vi "Phasor Compute SEPL v2.vi"(6 "Tick Length (0.02)":dbl=0.02, 8 "Error In":errorcluster, 9 "Compute Lifetime/Fraction Array":bool, 11 "Phasor Parameters":T4={"Display Parameters"={"# Points"=0, "Ramp Type"=enum."Linear", "Type of Series"=enum."1-Exp Decays", "Min tau"=0.0, "Max tau"=0.0, "Include 0"=FALSE, "Include Infinity"=FALSE}, "Phasor Parameters"={"Harmonic Frequency"=0.0, "Use f* = 1/D Frequency"=FALSE, "Calibrated Phasor"=FALSE, "Calibration Lifetime"=1e-09, "Phasor Calculation"=enum."Direct Sum", "SEPL Type"=enum."UC", "# Gates"=1.0, "Square Gate Width"=1e-09, "Show Ticks"=FALSE}, "Decay & IRF Parameters"={"Lifetime"=0.0, "IRF Offset"=0.0, "IRF Period"=0.0, "Normalized Decays"=FALSE, "IRF Model"=enum."Dirac", "IRF Parameter 1"=0.0}, "Gate Parameters"={"First Gate Start"=0.0, "Use Gate Center"=FALSE, "Gate Width"=0.0, "Gate Step"=0.0, "# Gates"=0.0, "Gate Type"=enum."Square", "Edge Width"=0.0, "Top Slope"=0.0, "Reversed Sawtooth?"=FALSE, "Analytical Computation"=FALSE, "Integration"=enum."Item 0", "Tolerance"=1.0, "# Steps"=1.0, "Type of User-defined Function"=enum."Gate", "Use Gate Step"=FALSE}, "Detector Parameters"={"Frames/Image"=0, "Gates/Frame"=0, "Bits/Frame"=0, "Multiplicity"=0, "Incident Signal"=0.0, "Poisson Signal"=FALSE}} {"Detector Parameters"."Frames/Image" min=1; "Detector Parameters"."Multiplicity" min=0; "Detector Parameters"."Bits/Frame" min=1; "Detector Parameters"."Gates/Frame" min=1; "Gate Parameters"."# Steps" min=0.0; "Gate Parameters"."Tolerance" min=0.0; "Gate Parameters"."Top Slope" min=0.0; "Gate Parameters"."Edge Width" min=0.0; "Gate Parameters"."Gate Step" min=0.0; "Gate Parameters"."# Gates" min=0.0 step=1.0; "Gate Parameters"."Gate Width" min=0.0; "Decay & IRF Parameters"."Lifetime" min=0.0; "Decay & IRF Parameters"."IRF Period" min=0.0; "Phasor Parameters"."Square Gate Width" min=0.0; "Phasor Parameters"."# Gates" min=0.0; "Phasor Parameters"."Calibration Lifetime" min=0.0; "Phasor Parameters"."Harmonic Frequency" min=0.0; "Display Parameters"."Min tau" min=0.0; "Display Parameters"."Max tau" min=0.0; "Display Parameters"."# Points" min=1 step=1}) -> (0 "Error Out":errorcluster, 1 "Plot Name":string, 2 "Plot Metadata":T3={"Lifetime/Fraction Array"=[], "Phasor Explorer Parameters"={"Display Parameters"={"# Points"=0, "Ramp Type"=enum."Linear", "Type of Series"=enum."1-Exp Decays", "Min tau"=0.0, "Max tau"=0.0, "Include 0"=FALSE, "Include Infinity"=FALSE}, "Phasor Parameters"={"Harmonic Frequency"=0.0, "Use f* = 1/D Frequency"=FALSE, "Calibrated Phasor"=FALSE, "Calibration Lifetime"=1e-09, "Phasor Calculation"=enum."Direct Sum", "SEPL Type"=enum."UC", "# Gates"=1.0, "Square Gate Width"=1e-09, "Show Ticks"=FALSE}, "Decay & IRF Parameters"={"Lifetime"=0.0, "IRF Offset"=0.0, "IRF Period"=0.0, "Normalized Decays"=FALSE, "IRF Model"=enum."Dirac", "IRF Parameter 1"=0.0}, "Gate Parameters"={"First Gate Start"=0.0, "Use Gate Center"=FALSE, "Gate Width"=0.0, "Gate Step"=0.0, "# Gates"=0.0, "Gate Type"=enum."Square", "Edge Width"=0.0, "Top Slope"=0.0, "Reversed Sawtooth?"=FALSE, "Analytical Computation"=FALSE, "Integration"=enum."Item 0", "Tolerance"=1.0, "# Steps"=1.0, "Type of User-defined Function"=enum."Gate", "Use Gate Step"=FALSE}, "Detector Parameters"={"Frames/Image"=0, "Gates/Frame"=0, "Bits/Frame"=0, "Multiplicity"=0, "Incident Signal"=0.0, "Poisson Signal"=FALSE}}, "Phase Lifetimes"=[], "Modulus Lifetimes"=[]} {"Phasor Explorer Parameters"."Detector Parameters"."Frames/Image" min=1; "Phasor Explorer Parameters"."Detector Parameters"."Multiplicity" min=0; "Phasor Explorer Parameters"."Detector Parameters"."Bits/Frame" min=1; "Phasor Explorer Parameters"."Detector Parameters"."Gates/Frame" min=1; "Phasor Explorer Parameters"."Gate Parameters"."# Steps" min=0.0; "Phasor Explorer Parameters"."Gate Parameters"."Tolerance" min=0.0; "Phasor Explorer Parameters"."Gate Parameters"."Top Slope" min=0.0; "Phasor Explorer Parameters"."Gate Parameters"."Edge Width" min=0.0; "Phasor Explorer Parameters"."Gate Parameters"."Gate Step" min=0.0; "Phasor Explorer Parameters"."Gate Parameters"."# Gates" min=0.0 step=1.0; "Phasor Explorer Parameters"."Gate Parameters"."Gate Width" min=0.0; "Phasor Explorer Parameters"."Decay & IRF Parameters"."Lifetime" min=0.0; "Phasor Explorer Parameters"."Decay & IRF Parameters"."IRF Period" min=0.0; "Phasor Explorer Parameters"."Phasor Parameters"."Square Gate Width" min=0.0; "Phasor Explorer Parameters"."Phasor Parameters"."# Gates" min=0.0; "Phasor Explorer Parameters"."Phasor Parameters"."Calibration Lifetime" min=0.0; "Phasor Explorer Parameters"."Phasor Parameters"."Harmonic Frequency" min=0.0; "Phasor Explorer Parameters"."Display Parameters"."Min tau" min=0.0; "Phasor Explorer Parameters"."Display Parameters"."Max tau" min=0.0; "Phasor Explorer Parameters"."Display Parameters"."# Points" min=1 step=1}, 3 "Single Exponential Phasor Plot":cluster{"Array":dbl[], "Array":dbl[]}, 4 "Tick Label Data":T1[](array[typedef]), 5 "Phasor Calculation":T8, 7 "CPU (s)":dbl)   [LabVIEW 2021, in "Phasor.lvlib"]
uses:
  Phasor.lvlib
  Phasor SEPL Parameters.ctl
  Phasor Explorer Display Parameters.ctl
  Phasor Type of Series.ctl
  Phasor Explorer Phasor Parameters.ctl
  Phasor Calculation Type.ctl
  Phasor SEPL Type.ctl
  Phasor Explorer Decay Parameters.ctl
  Phasor IRF Model.ctl
  Phasor Explorer Gate Parameters.ctl
  Phasor Gate Type.ctl
  Phasor Type of User-defined Function.ctl
  Phasor Explorer Detector Parameters.ctl
  Phasor Explorer Phasor Plot Info.ctl
  Phasor SEPL Tick Data.ctl
  Phasor (g, s).ctl
  Phasor Calibration Data.ctl
  Phasor L_N[W] Parameters.ctl
  ba521b30-8e21-40a0-90b4-9632ea6a7fe5.vi
  Phasor Explorer.lvlib
  Time/Time.lvlib
panel:
  out "# Rejected Pairs":i32
  out "Lifetime/Fraction Array":dbl[](array[numeric])
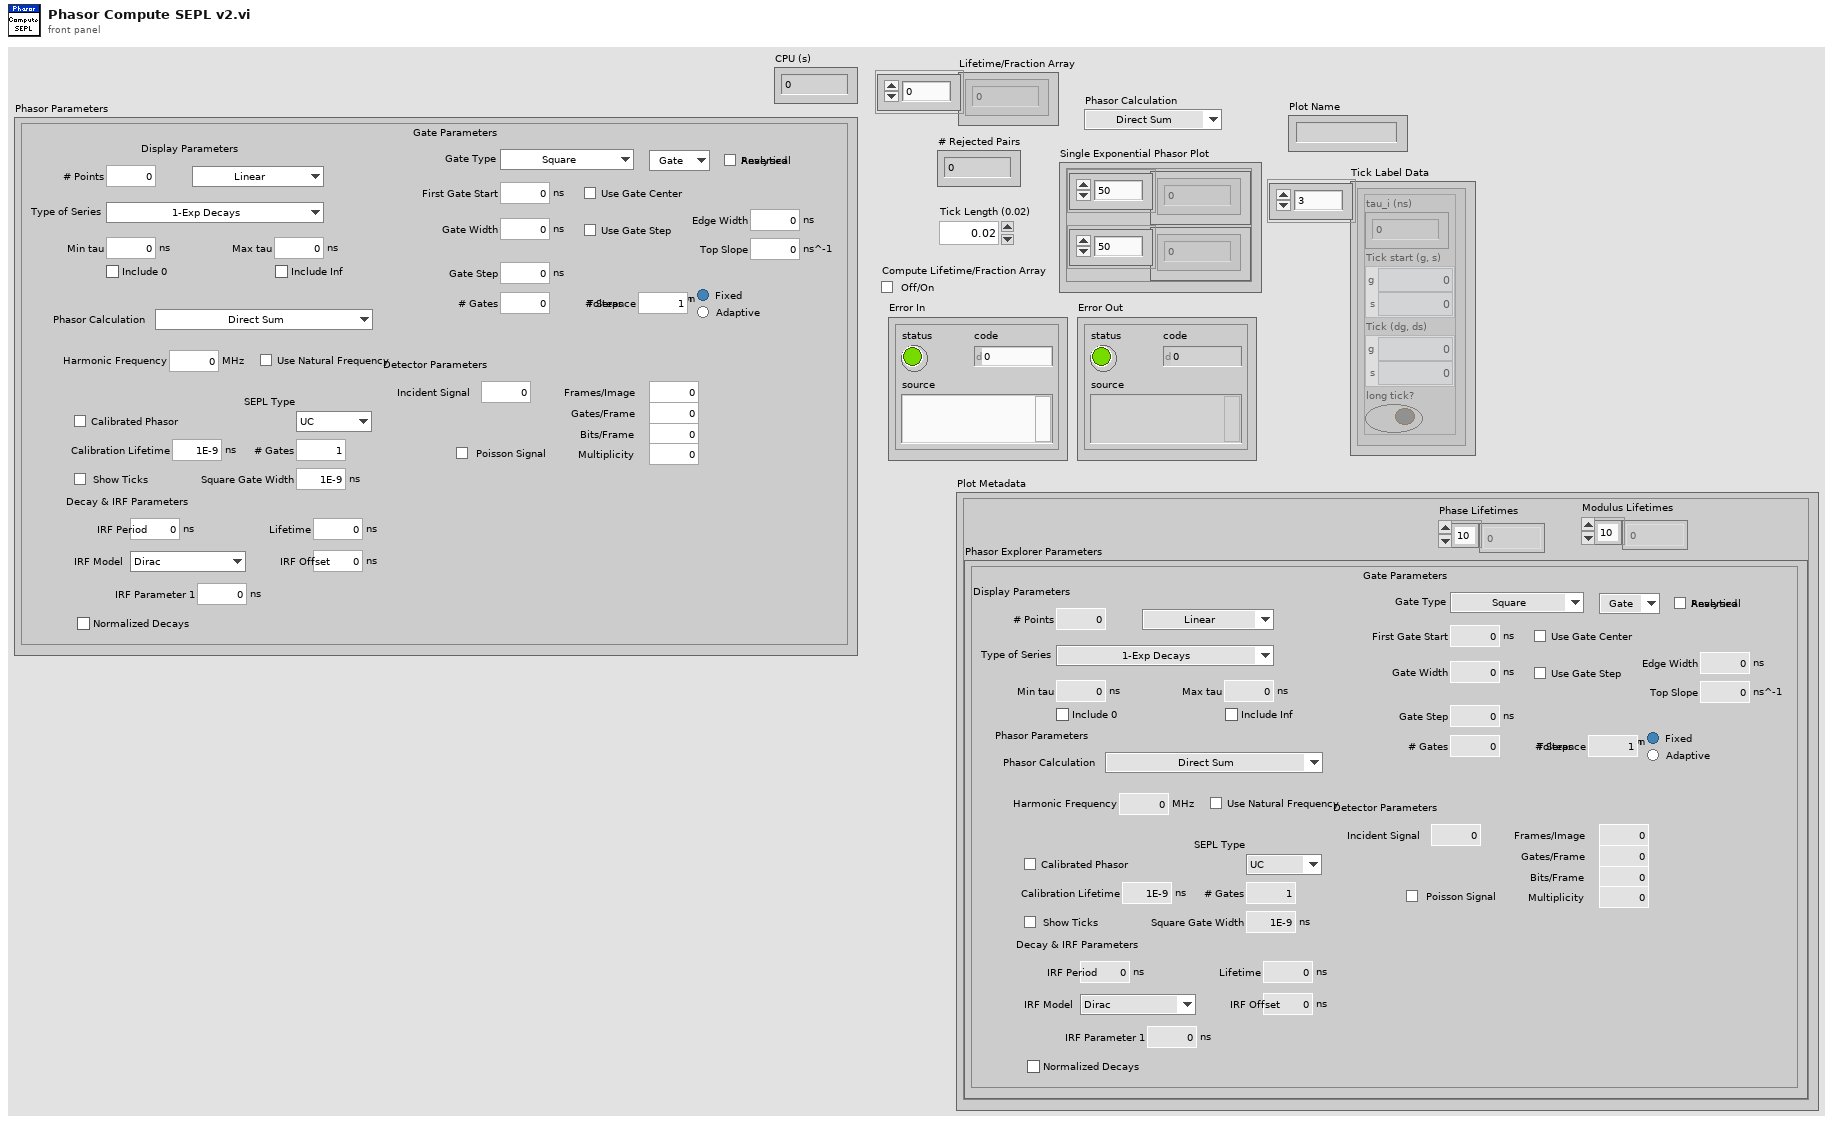
[diagram p1: front panel]
types:
  T1 = typedef "Phasor.lvlib/Phasor SEPL Tick Data.ctl" = cluster{"tau_i (ns)":dbl, "Tick start (g, s)":T2, "Tick (dg, ds)":T2, "long tick?":bool}
  T2 = typedef "Phasor.lvlib/Phasor (g, s).ctl" = cluster{"g":dbl, "s":dbl}
  T3 = typedef "Phasor Explorer.lvlib/Phasor Explorer Phasor Plot Info.ctl" = cluster{"Lifetime/Fraction Array":dbl[], "Phasor Explorer Parameters":T4, "Phase Lifetimes":dbl[], "Modulus Lifetimes":dbl[]}
  T4 = typedef "Phasor.lvlib/Phasor SEPL Parameters.ctl" = cluster{"Display Parameters":T5, "Phasor Parameters":T7, "Decay & IRF Parameters":T10, "Gate Parameters":T12, "Detector Parameters":T15}
  T5 = typedef "Phasor Explorer.lvlib/Phasor Explorer Display Parameters.ctl" = cluster{"# Points":i32, "Ramp Type":enum16{"Linear", "Logarithmic"}, "Type of Series":T6, "Min tau":dbl[unit], "Max tau":dbl[unit], "Include 0":bool, "Include Infinity":bool}
  T6 = typedef "Phasor.lvlib/Phasor Type of Series.ctl" = enum16{"1-Exp Decays", "Linear Combination of 1-Exp"}
  T7 = typedef "Phasor Explorer.lvlib/Phasor Explorer Phasor Parameters.ctl" = cluster{"Harmonic Frequency":dbl[unit], "Use f* = 1/D Frequency":bool, "Calibrated Phasor":bool, "Calibration Lifetime":dbl[unit], "Phasor Calculation":T8, "SEPL Type":T9, "# Gates":dbl, "Square Gate Width":dbl[unit], "Show Ticks":bool}
  T8 = typedef "Phasor.lvlib/Phasor Calculation Type.ctl" = enum16{"Direct Sum", "Analytical Formula"}
  T9 = typedef "Phasor.lvlib/Phasor SEPL Type.ctl" = enum16{"UC", "L_N", "L_N[W]", "L_X"}
  T10 = typedef "Phasor Explorer.lvlib/Phasor Explorer Decay Parameters.ctl" = cluster{"Lifetime":dbl[unit], "IRF Offset":dbl[unit], "IRF Period":dbl[unit], "Normalized Decays":bool, "IRF Model":T11, "IRF Parameter 1":dbl[unit]}
  T11 = typedef "Phasor.lvlib/Phasor IRF Model.ctl" = enum16{"Dirac", "Exponential"}
  T12 = typedef "Phasor Explorer.lvlib/Phasor Explorer Gate Parameters.ctl" = cluster{"First Gate Start":dbl[unit], "Use Gate Center":bool, "Gate Width":dbl[unit], "Gate Step":dbl[unit], "# Gates":dbl, "Gate Type":T13, "Edge Width":dbl[unit], "Top Slope":dbl[unit], "Reversed Sawtooth?":bool, "Analytical Computation":bool, "Integration":enum32{"Item 0", "Item 1"}, "Tolerance":dbl, "# Steps":dbl, "Type of User-defined Function":T14, "Use Gate Step":bool}
  T13 = typedef "Phasor.lvlib/Phasor Gate Type.ctl" = enum16{"Square", "Finite Edge Square", "Finite Edge, Tilted Top Square", "Triangle", "Sawtooth", "User-defined"}
  T14 = typedef "Phasor.lvlib/Phasor Type of User-defined Function.ctl" = enum16{"Gate", "IRF"}
  T15 = typedef "Phasor Explorer.lvlib/Phasor Explorer Detector Parameters.ctl" = cluster{"Frames/Image":i32, "Gates/Frame":i32, "Bits/Frame":i32, "Multiplicity":i32, "Incident Signal":dbl, "Poisson Signal":bool}
  T16 = typedef "Phasor.lvlib/Phasor L_N[W] Parameters.ctl" = cluster{"Laser Period":dbl[unit], "Gate Width":dbl[unit], "Gate Step":dbl[unit], "Harmonic frequency":dbl[unit], "IRF offset":dbl[unit], "# Gates":dbl}
  T17 = typedef "Phasor.lvlib/Phasor Calibration Data.ctl" = cluster{"jw":cxt, "Uncalibrated Phasor":cxt, "Calibrated Phasor":cxt, "Calibrated Phasor?":bool, "Calibration Lifetime":ext}
  T18 = typedef "Phasor.lvlib/Phasor Gate Definitions.ctl" = cluster{"First Gate: t1":ext, "Gate Width: W":ext, "Gate Step: d":ext, "# Gates: G":ext, "Use Gate Center":bool, "Frames/Image: F":i32, "Gates/Frame: L":i32, "Bits/Frame: q":i32, "Multiplicity: p":i32, "Gate Type":T13, "Gate Edge s":ext, "Gate Top Slope":ext, "Reversed Sawtooth?":bool, "Computation":bool, "User-defined Gate":T19, "Tolerance":ext, "Integration":enum32{"Item 0", "Item 1"}, "# Steps":ext, "Type of User-defined Function":enum32{"Gate", "IRF"}}
  T19 = typedef "XY Graph Add-Ons.lvlib/XY Plot Data.ctl" = cluster{"X Array":dbl[], "Y Array":dbl[]}
  T20 = typedef "Phasor.lvlib/Phasor Decay Definiton.ctl" = cluster{"offset: t0":ext, "period: T":ext, "lifetime: tau":ext, "Incident Signal: I":ext, "Normalized Decays":bool, "IRF Model":T11, "IRF Parameter 1":ext, "Poisson Signal":bool}
  T21 = cluster{"Numeric Control":ext, "Numeric Control":ext}
  T22 = cluster{"Calibrated g Array out":ext[], "Calibrated s Array out":ext[]}
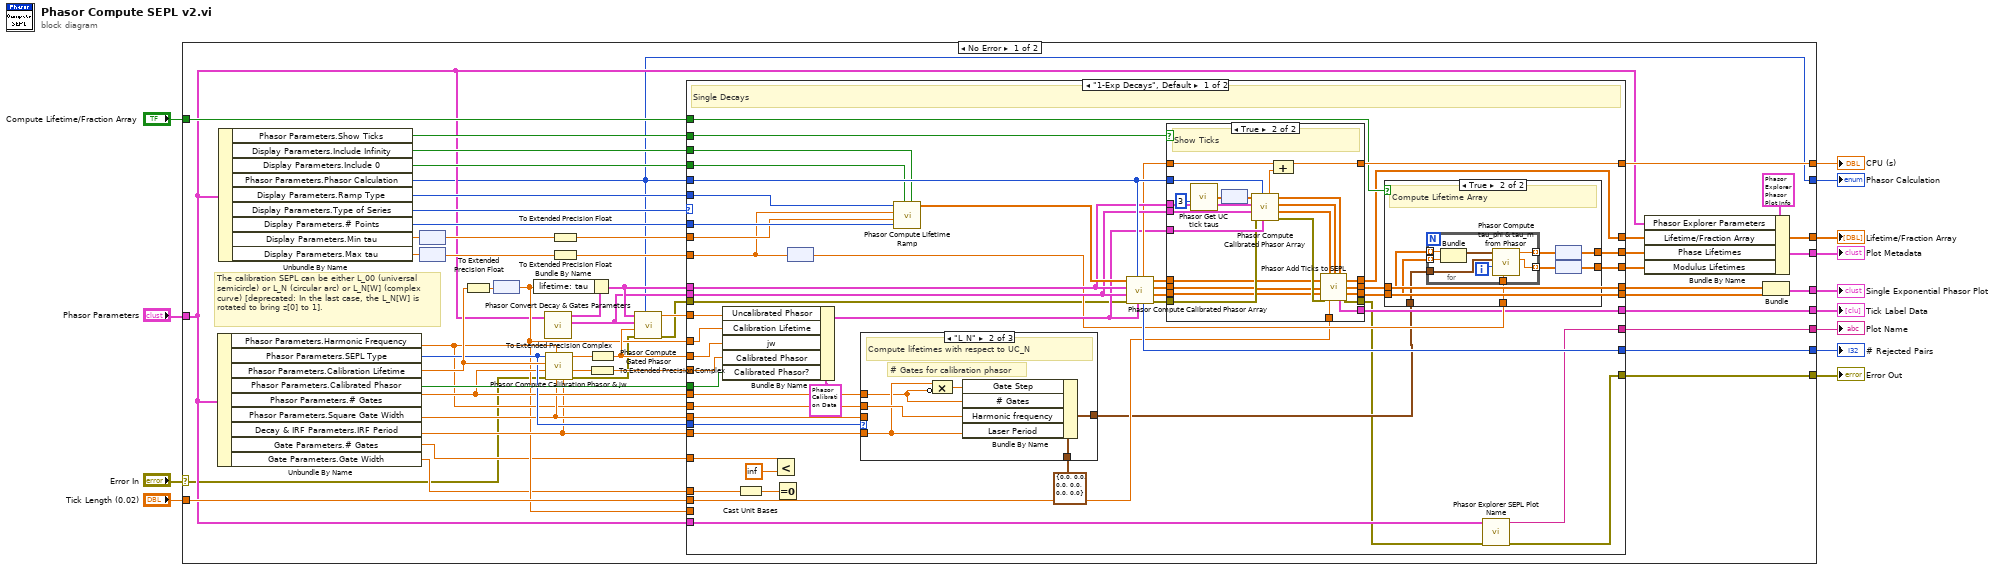
[diagram p0: block diagram]
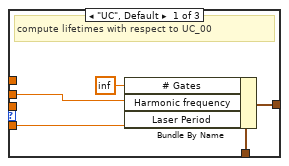
[diagram p4: hidden frame]
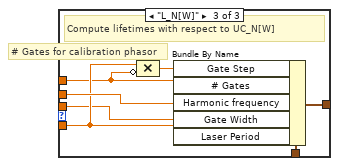
[diagram p5: hidden frame]
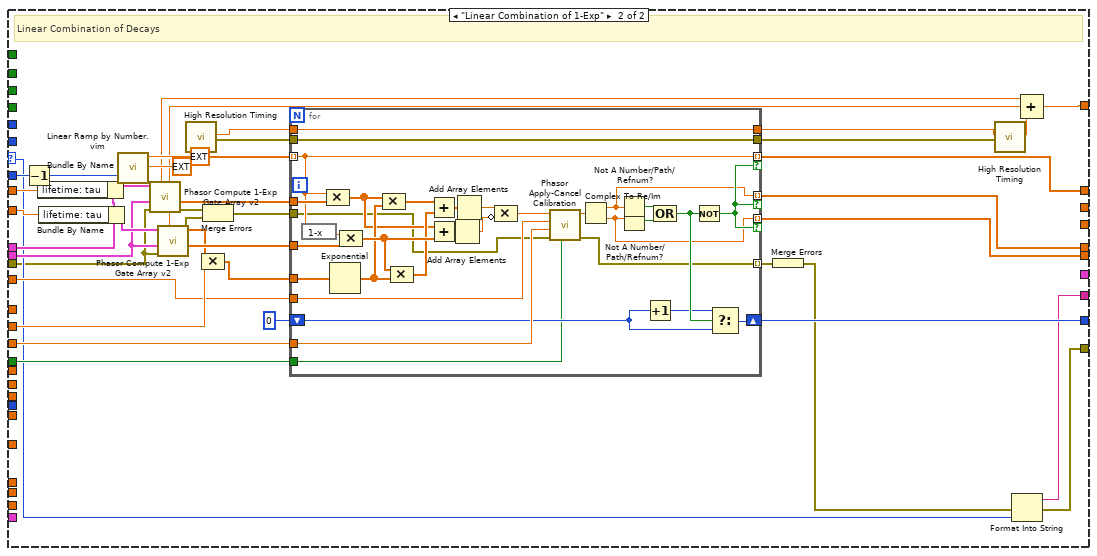
[diagram p6: hidden frame]
diagram:
  n1 = case shown="No Error" "Error In" {
    selector: "Error In" -> [w17 w251]
    tunnel: "Phasor Parameters" -> [w18 _]
    tunnel: [w58 _] -> w12
    tunnel: [w30 w251] -> w10
    tunnel: [w39 _] -> w9
    tunnel: [w14 _] -> w8
    tunnel: [w29 _] -> w7
    tunnel: [w45 _] -> w6
    tunnel: [w34 _] -> w5
    tunnel: [w32 _] -> w4
    tunnel: "Compute Lifetime/Fraction Array" -> [w28 _]
    tunnel: "Tick Length (0.02)" -> [w27 _]
    tunnel: [w26 _] -> w1
    frame No Error {
      # "The calibration SEPL can be either L_00 (universal semicircle) or L_N (circular arc) or L_N[W] (complex curve) [deprecated: In the last case, the L_N[W] is rotated to bring z[0] to 1]."
      n2 = Unbundle By Name(w18) -> ("Phasor Parameters.Harmonic Frequency"=w23:dbl[unit], "Phasor Parameters.SEPL Type"=w35:T9, "Phasor Parameters.Calibration Lifetime"=w41:dbl[unit], "Phasor Parameters.Calibrated Phasor"=w50:bool, "Phasor Parameters.# Gates"=w25:dbl, "Phasor Parameters.Square Gate Width"=w24:dbl[unit], "Decay & IRF Parameters.IRF Period"=w22:dbl[unit], "Gate Parameters.# Gates"=w20:dbl, "Gate Parameters.Gate Width"=w19:dbl[unit])
      n3 = Unbundle By Name(w18) -> ("Phasor Parameters.Show Ticks"=w33:bool, "Display Parameters.Include Infinity"=w48:bool, "Display Parameters.Include 0"=w49:bool, "Phasor Parameters.Phasor Calculation"=w14:T8, "Display Parameters.Ramp Type"=w57:enum16{"Linear", "Logarithmic"}, "Display Parameters.Type of Series"=w53:T6, "Display Parameters.# Points"=w31:i32, "Display Parameters.Min tau"=w59:dbl[unit], "Display Parameters.Max tau"=w64:dbl[unit])
      n4 = node(w59) -> (w55:dbl)
      n5 = node(w64) -> (w54:dbl)
      n6 = To Extended Precision Float(1:w41) -> (0:w43:ext[unit])
      n7 = node(w43) -> (w21:ext)
      n8 = call "Phasor Convert Decay & Gates Parameters.vi"("Phasor Parameters"=w18) -> ("Gates Definitions"=w51:T18, "Decay Definition"=w52:T20)  [unwired: 9 in]
      n9 = Bundle By Name(cluster=w52, "lifetime: tau"=w21) -> (w60:T20)
      n10 = call "Phasor Compute Calibration Phasor & jw.vi"("Laser Period"=w22, "Gate Width"=w24, "Harmonic frequency"=w23, "Error In"=w17, "# Gates"=w25, "Calibration Lifetime"=w41, "Calibration Phasor Type"=w35) -> ("Error Out"=w16:errorcluster, "z (tau_cal)"=w36:cdb, "i 2 pi f (GHz)"=w56:cdb)  [unwired: 2 in]
      n11 = To Extended Precision Float(1:w55) -> (0:w47:ext)
      n12 = To Extended Precision Float(1:w54) -> (0:w46:ext)
      n13 = To Extended Precision Complex(1:w36) -> (0:w44:cxt)
      n14 = To Extended Precision Complex(1:w56) -> (0:w42:cxt)
      n15 = call "Phasor Compute Gated Phasor.vi"("Phasor Calculation Type"=w14, "Error In"=w16, "j 2 pi f"=w42, "Gates Definitions"=w51, "Decay Definition"=w60) -> ("Error Out"=w15:errorcluster, "phasor"=w61:cxt)  [unwired: 4 in, 1 out]
      n16 = case shown="\"1-Exp Decays\", Default" w53 {
        selector: w53 -> [_ w181]
        tunnel: [w89 w197] -> w63
        tunnel: [w88 w196] -> w62
        tunnel: w50 -> [w69 w205]
        tunnel: w61 -> [w114 w203]
        tunnel: w60 -> [w98 w217]
        tunnel: w51 -> [w97 w213]
        tunnel: w42 -> [w111 w207]
        tunnel: w44 -> [w113 w204]
        tunnel: w47 -> [w82 w218]
        tunnel: w46 -> [w81 w216]
        tunnel: w57 -> [w84 _]
        tunnel: w21 -> [w110 _]
        tunnel: w14 -> [w100 _]
        tunnel: [w71 w198] -> w39
        tunnel: [w65 w178] -> w30
        tunnel: w49 -> [w86 _]
        tunnel: w48 -> [w85 _]
        tunnel: [w108 w199] -> w45
        tunnel: [w106 _] -> w38
        tunnel: [w107 _] -> w37
        tunnel: w35 -> [w78 _]
        tunnel: w23 -> [w104 _]
        tunnel: w22 -> [w103 _]
        tunnel: w25 -> [w102 _]
        tunnel: [w95 w189] -> w34
        tunnel: w24 -> [w101 _]
        tunnel: w33 -> [w99 _]
        tunnel: w31 -> [w83 w184]
        tunnel: [w68 w182] -> w29
        tunnel: w28 -> [w80 _]
        tunnel: w27 -> [w75 _]
        tunnel: [w79 _] -> w26
        tunnel: w21 -> [_ _]
        tunnel: w20 -> [w77 _]
        tunnel: w19 -> [w73 _]
        tunnel: w18 -> [w70 _]
        tunnel: w15 -> [w67 w180]
        frame "1-Exp Decays", Default {
          # "Single Decays"
          n17 = Bundle By Name(cluster=T17 {"jw"=0.0+0.0i, "Uncalibrated Phasor"=0.0+0.0i, "Calibrated Phasor"=0.0+0.0i, "Calibrated Phasor?"=FALSE, "Calibration Lifetime"=0.0} ("output cluster"), "Uncalibrated Phasor"=w114, "Calibration Lifetime"=w110, "jw"=w111, "Calibrated Phasor"=w113, "Calibrated Phasor?"=w69) -> (w91:T17)
          n18 = Cast Unit Bases(0:w73) -> (2:w72:dbl)  [unwired: 1 in]
          n19 = Less?(x=w77, y=inf) -> ()  [unwired: 1 out]
          n20 = Equal To 0?(x=w72) -> ()  [unwired: 1 out]
          n21 = node(w81) -> (w87:ext[unit])
          n22 = case shown="\"L_N\"" w78 {
            tunnel: [w164 w170 w177] -> w74
            tunnel: T16 {"Laser Period"=0.0, "Gate Width"=0.0, "Gate Step"=0.0, "Harmonic frequency"=0.0, "IRF offset"=0.0, "# Gates"=0.0} ("Phasor UCN[W] Parameters") -> [w162 w169 w176]
            tunnel: w104 -> [w161 w168 w175]
            tunnel: w103 -> [w160 w167 w174]
            tunnel: w102 -> [_ w165 w172]
            tunnel: w101 -> [_ _ w171]
            frame "UC", Default {
              # "compute lifetimes with respect to UC_00"
              n23 = Bundle By Name(cluster=w162, "# Gates"=inf ("Gate Parameters.# Gates"), "Harmonic frequency"=w161, "Laser Period"=w160) -> (w164:T16)
            }
            frame "L_N" {
              # "# Gates for calibration phasor"
              # "Compute lifetimes with respect to UC_N"
              n24 = Compound Arithmetic op=MULTIPLY(w167, invert w165) -> (w166:dbl[unit])
              n25 = Bundle By Name(cluster=w169, "Gate Step"=w166, "# Gates"=w165, "Harmonic frequency"=w168, "Laser Period"=w167) -> (w170:T16)
            }
            frame "L_N[W]" {
              # "# Gates for calibration phasor"
              # "Compute lifetimes with respect to UC_N[W]"
              n26 = Compound Arithmetic op=MULTIPLY(w174, invert w172) -> (w173:dbl[unit])
              n27 = Bundle By Name(cluster=w176, "Gate Step"=w173, "# Gates"=w172, "Harmonic frequency"=w175, "Gate Width"=w171, "Laser Period"=w174) -> (w177:T16)
            }
          }
          n28 = call "Phasor Compute Lifetime Ramp.vi"("Include Infinity"=w85, "Include 0"=w86, "# Points"=w83, "Min Tau"=w82, "Max Tau"=w81, "Ramp Type"=w84) -> ("Lifetime Ramp"=w109:ext[])  [unwired: 5 in]
          n29 = call "Phasor Compute Calibrated Phasor Array.vi"("Phasor Calibration Data"=w91, "Phasor Calculation"=w100, "Error In"=w67, "Gates Definitions"=w97, "Decay Definition"=w98, "Lifetime Array"=w109) -> ("Error Out"=w90:errorcluster, "Calibrated s Array"=w92:ext[], "Calibrated g Array"=w93:ext[], "True Lifetime Array"=w94:ext[], "# Rejected Pairs"=w108:i32, "CPU (s)"=w96:dbl)
          n30 = case shown="True" w99 {
            tunnel: w100 -> [_ w159]
            tunnel: w98 -> [_ w158]
            tunnel: w97 -> [_ w157]
            tunnel: [w134 w148] -> w66
            tunnel: w96 -> [w135 w156]
            tunnel: [w135 w154] -> w95
            tunnel: w94 -> [w133 w146]
            tunnel: w93 -> [w132 w145]
            tunnel: w92 -> [w131 w144]
            tunnel: w91 -> [_ w151]
            tunnel: w90 -> [w134 w150]
            tunnel: [w133 w143] -> w71
            tunnel: [w132 w142] -> w89
            tunnel: [w131 w141] -> w88
            tunnel: w75 -> [_ w138]
            tunnel: [_ w137] -> w79
            frame False {
            }
            frame True {
              # "Show Ticks"
              n31 = call "Phasor Get UC tick taus.vi"("# Decades (4: 10 ps - 900 ns)"=3) -> ("Array of taus"=w153:dbl[unit][])  [unwired: 7 in]
              n32 = node(w153) -> (w152:dbl[])
              n33 = call "Phasor Compute Calibrated Phasor Array.vi"("Phasor Calibration Data"=w151, "Phasor Calculation"=w159, "Error In"=w150, "Gates Definitions"=w157, "Decay Definition"=w158, "Lifetime Array"=w152) -> ("Error Out"=w149:errorcluster, "Calibrated s Array"=w140:ext[], "Calibrated g Array"=w139:ext[], "True Lifetime Array"=w147:ext[], "CPU (s)"=w155:dbl)  [unwired: 1 out]
              n34 = Compound Arithmetic op=ADD(w156, w155) -> (w154:dbl)
              n35 = call "Phasor Add Ticks to SEPL.vi"("Ticks Calibrated s's"=w140, "Ticks Calibrated g's"=w139, "Ticks Lifetimes"=w147, "Lifetime Array in"=w146, "Calibrated g Array in"=w145, "Calibrated s Array in"=w144, "error in (no error)"=w149, "Tick Length"=w138) -> ("Lifetime Array out"=w143:ext[], "Calibrated g Array out"=w142:ext[], "Calibrated s Array out"=w141:ext[], "Tick Labels (g,s))"=w137:T1[], "error out"=w148:errorcluster)  [unwired: 3 in]
            }
          }
          n36 = case shown="True" w80 {
            tunnel: [_ w120] -> w107
            tunnel: [_ w119] -> w106
            tunnel: w74 -> [_ w118]
            tunnel: w89 -> [_ w117]
            tunnel: w88 -> [_ w116]
            tunnel: w87 -> [_ w115]
            frame False {
            }
            frame True {
              # "Compute Lifetime Array"
              n37 = for {
                tunnel: w115 -> [w124]
                tunnel: w118 -> [w125]
                tunnel: w117 -> [w128] mode=indexing
                tunnel: w116 -> [w127] mode=indexing
                tunnel: [w130] -> w122 mode=indexing
                tunnel: [w129] -> w121 mode=indexing
                i -> [w123]
                n38 = Bundle("Numeric Control"=w128, "Numeric Control"=w127) -> (w126:T21)  [unwired: 1 in]
                n39 = call "Phasor Compute tau_phi & tau_m from Phasor.vi"("max tau"=w124, "Call # (0)"=w123, "Phasor L_N[W] Parameters"=w125, "Phasor"=w126) -> ("tau_m"=w130:dbl[unit], "tau_ph"=w129:dbl[unit])  [unwired: 5 in, 1 out]
              }
              n40 = node(w121) -> (w120:dbl[])
              n41 = node(w122) -> (w119:dbl[])
            }
          }
          n42 = call "Phasor Explorer SEPL Plot Name.vi"("Error In"=w66, "Phasor Parameters"=w70) -> ("Error Out"=w65:errorcluster, "SEPL Plot Name"=w68:string)  [unwired: 8 in]
        }
        frame "Linear Combination of 1-Exp" {
          # "Linear Combination of Decays"
          n43 = Decrement(x=w184) -> (x-1=w183:i32)
          n44 = Bundle By Name(cluster=w217, "lifetime: tau"=w218) -> (w215:T20)
          n45 = Bundle By Name(cluster=w217, "lifetime: tau"=w216) -> (w214:T20)
          n46 = call "Linear Ramp by Number.vim"("# Steps (1)"=w183, "End (1)"=ext 1.0 ("Max"), "Start (0)"=ext 0.0 ("Min")) -> ("Ramp"=w200:ext[])  [unwired: 6 in, 2 out]
          n47 = call "Phasor Compute 1-Exp Gate Array v2.vi"("Error In"=w180, "Gates Definitions"=w213, "Decay Definition"=w215) -> ("Error Out"=w202:errorcluster, "Gate Image Array"=w210:ext[], "CPU (s)"=w188:dbl)  [unwired: 4 in, 2 out]
          n48 = call "Phasor Compute 1-Exp Gate Array v2.vi"("Error In"=w180, "Gates Definitions"=w213, "Decay Definition"=w214) -> ("Error Out"=w201:errorcluster, "Gate Image Array"=w209:ext[], "t Array"=w208:ext[], "CPU (s)"=w187:dbl)  [unwired: 4 in, 1 out]
          n49 = call "High Resolution Timing.vi"() -> ("elapsed (relative) seconds"=w192:dbl, "Error Out"=w194:errorcluster)  [unwired: 17 in, 1 out]
          n50 = Compound Arithmetic op=MULTIPLY(w208, w207) -> (w206:cxt[])
          n51 = Merge Errors(w202, w201) -> (w186:errorcluster)
          n52 = for {
            tunnel: w210 -> [w250]
            tunnel: w209 -> [w249]
            tunnel: w200 -> [w230] mode=indexing
            tunnel: w206 -> [w248]
            tunnel: [w226] -> w196 mode=indexing if=w229
            tunnel: [w225] -> w197 mode=indexing if=w229
            tunnel: w205 -> [w221]
            tunnel: w204 -> [w235]
            tunnel: w203 -> [w234]
            tunnel: [w230] -> w198 mode=indexing if=w229
            shift-right: [w228] -> w199
            shift-left: 0 -> [w227]
            tunnel: w194 -> [w223]
            tunnel: [w223] -> w193
            tunnel: w192 -> [w222]
            tunnel: [w222] -> w191
            tunnel: w186 -> [w220]
            tunnel: [w219] -> w185 mode=indexing
            n53 = expression code="1-x"(w230) -> (w245:ext)
            n54 = Compound Arithmetic op=MULTIPLY(w230, w250) -> (w240:ext[])
            n55 = Exponential(1:w248) -> (0:w246:cxt[])
            n56 = Compound Arithmetic op=MULTIPLY(w245, w249) -> (w247:ext[])
            n57 = Compound Arithmetic op=MULTIPLY(w240, w246) -> (w244:cxt[])
            n58 = Compound Arithmetic op=MULTIPLY(w247, w246) -> (w243:cxt[])
            n59 = Add(x=w244, y=w243) -> (x+y=w242:cxt[])
            n60 = Add(x=w240, y=w247) -> (x+y=w241:ext[])
            n61 = Add Array Elements(numeric array=w241) -> (sum=w238:ext)
            n62 = Add Array Elements(numeric array=w242) -> (sum=w239:cxt)
            n63 = Compound Arithmetic op=MULTIPLY(w239, invert w238) -> (w237:cxt)
            n64 = call "Phasor Apply-Cancel Calibration.vi"("Calibrated Phasor"=w221, "Error In"=w220, "Target Phasor"=w235, "Calibration Phasor"=w234, "Phasor in"=w237) -> ("Error Out"=w219:errorcluster, "Phasor out"=w236:cxt)  [unwired: 5 in]
            n65 = Complex To Re/Im(x + iy=w236) -> (x=w225:ext, y=w226:ext)
            n66 = Not A Number/Path/Refnum?(number/path/refnum=w225) -> (NaN/Path/Refnum?=w224:bool)
            n67 = Not A Number/Path/Refnum?(number/path/refnum=w226) -> (NaN/Path/Refnum?=w233:bool)
            n68 = Increment(x=w227) -> (x+1=w231:i32)
            n69 = Compound Arithmetic op=OR(w224, w233) -> (w232:bool)
            n70 = Not(x=w232) -> (.not. x?=w229:bool)
            n71 = Select(t=w231, s=w232, f=w227) -> (s? t:f=w228:i32)
          }
          n72 = Merge Errors(w185) -> (w179:errorcluster)
          n73 = call "High Resolution Timing.vi"("relative seconds (NaN)"=w191, "Error In"=w193) -> ("elapsed (relative) seconds"=w190:dbl)  [unwired: 15 in, 2 out]
          n74 = Format Into String(error in=w179, w181) -> (resulting string=w182:string, error out=w178:errorcluster)  [unwired: 2 in]
          n75 = Compound Arithmetic op=ADD(w188, w187, w190) -> (w189:dbl)
        }
      }
      n76 = Bundle By Name(cluster=T3 {"Lifetime/Fraction Array"=[], "Phasor Explorer Parameters"={"Display Parameters"={"# Points"=0, "Ramp Type"=enum."Linear", "Type of Series"=enum."1-Exp Decays", "Min tau"=0.0, "Max tau"=0.0, "Include 0"=FALSE, "Include Infinity"=FALSE}, "Phasor Parameters"={"Harmonic Frequency"=0.0, "Use f* = 1/D Frequency"=FALSE, "Calibrated Phasor"=FALSE, "Calibration Lifetime"=1e-09, "Phasor Calculation"=enum."Direct Sum", "SEPL Type"=enum."UC", "# Gates"=1.0, "Square Gate Width"=1e-09, "Show Ticks"=FALSE}, "Decay & IRF Parameters"={"Lifetime"=0.0, "IRF Offset"=0.0, "IRF Period"=0.0, "Normalized Decays"=FALSE, "IRF Model"=enum."Dirac", "IRF Parameter 1"=0.0}, "Gate Parameters"={"First Gate Start"=0.0, "Use Gate Center"=FALSE, "Gate Width"=0.0, "Gate Step"=0.0, "# Gates"=0.0, "Gate Type"=enum."Square", "Edge Width"=0.0, "Top Slope"=0.0, "Reversed Sawtooth?"=FALSE, "Analytical Computation"=FALSE, "Integration"=enum."Item 0", "Tolerance"=1.0, "# Steps"=1.0, "Type of User-defined Function"=enum."Gate", "Use Gate Step"=FALSE}, "Detector Parameters"={"Frames/Image"=0, "Gates/Frame"=0, "Bits/Frame"=0, "Multiplicity"=0, "Incident Signal"=0.0, "Poisson Signal"=FALSE}}, "Phase Lifetimes"=[], "Modulus Lifetimes"=[]} ("Phasor Graph Plot Info"), "Phasor Explorer Parameters"=w18, "Lifetime/Fraction Array"=w39, "Phase Lifetimes"=w37, "Modulus Lifetimes"=w38) -> (w32:T3)
      n77 = Bundle("Calibrated g Array out"=w63, "Calibrated s Array out"=w62) -> (w58:T22)  [unwired: 1 in]
    }
    frame Error {
    }
  }
  "Error Out" <- w10
  "Single Exponential Phasor Plot" <- w12
  "Lifetime/Fraction Array" <- w9
  "Phasor Calculation" <- w8
  "Plot Name" <- w7
  "# Rejected Pairs" <- w6
  "CPU (s)" <- w5
  "Plot Metadata" <- w4
  "Tick Label Data" <- w1
